vi "Dialog Tester - Preempt.vi"() -> ()   [LabVIEW 2021]
doc: "<b>TEST VI</b> checking the pre-empt action for pop up types"
uses:
  a07ed418-7f18-49d3-b4e5-936e803124ba.vi
  3f576889-9c36-41da-af72-f2da2302e1a7.vi
  ad5c8732-6e62-4ff5-afd9-587a057d3cc7.vi
  5b332a5c-591b-4519-aea1-c482ff36093b.vi
  34588afc-315a-47d8-a701-ee64ae2e0537.vi
  ae7c03dc-1e40-4bc6-b034-dfda178a26ad.vi
  d50a1210-0545-4c1a-9356-5886067c6458.vi
  aeec75d7-a6fb-4d61-b6af-3d1469a3ba41.vi
  6fc38696-eeba-4556-84b5-67169f5a97e1.vi
  54b3774a-3740-4b7d-aaf4-c8348b3dcf84.vi
  f0ad3a18-8d1f-4dec-8074-68e03ac96f8e.vi
  cba20e50-060c-4cef-b2cd-495110a6043b.vi
  Standard/Input (DBL)/Input (DBL).lvclass
  Standard/Input (I32)/Input (I32).lvclass
  Standard/Input (String)/Input (String).lvclass
  Standard/Timeout/Timeout.lvclass
  Standard/Timeout One Button/Timeout One Button.lvclass
  Standard/Timeout Two Button/Timeout Two Button.lvclass
  Standard/Two Button/Two Button.lvclass
  Popup/Popup.lvclass
panel:
  out "Two-Button T.O. Choice? - val":bool
  out "Two-Button Choice? - val":bool
  out "Input Value (String - val)":string
  out "Input Value (I32 - val)":i32
  out "Input Value (DBL - close)":dbl
  out "Two-Button T.O. Choice? - close":bool
  out "Two-Button Choice? - close":bool
  out "Input Value (String - close)":string
  out "Input Value (I32 - close)":i32
  out "Input Value (DBL - val)":dbl
  out "iteration":i32
  in  "Error In":errorcluster
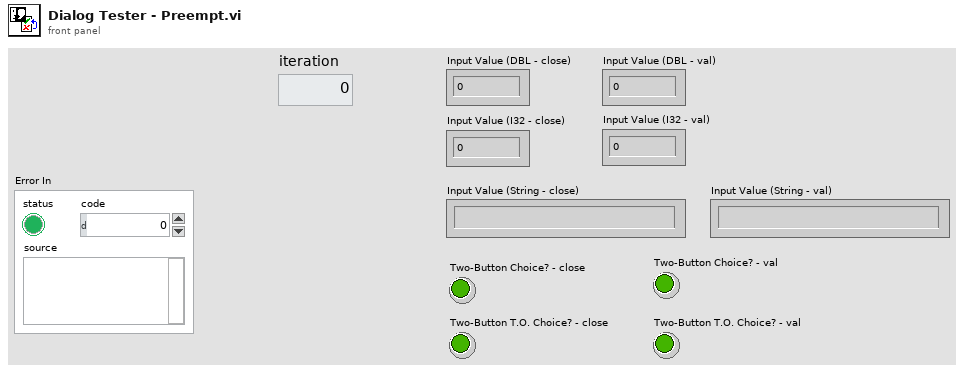
[diagram p1: front panel]
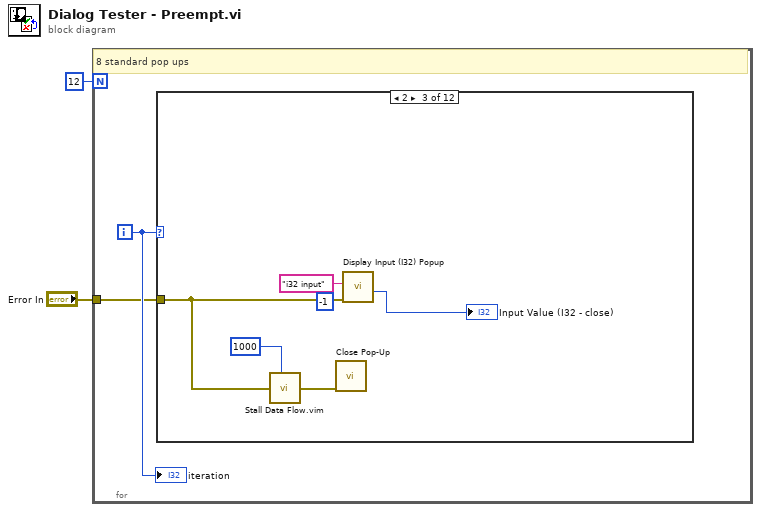
[diagram p0: block diagram]
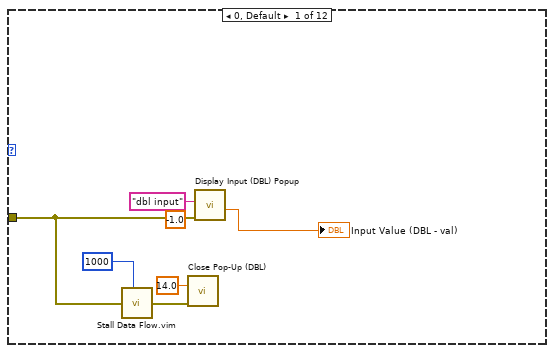
[diagram p2: hidden frame]
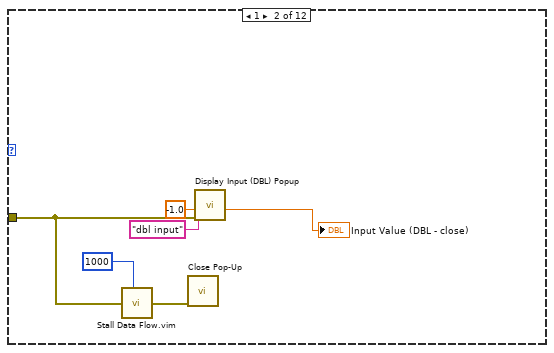
[diagram p3: hidden frame]
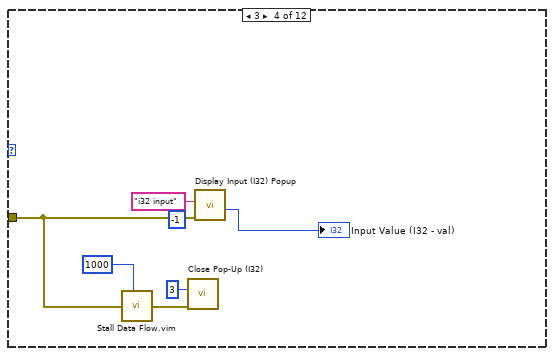
[diagram p4: hidden frame]
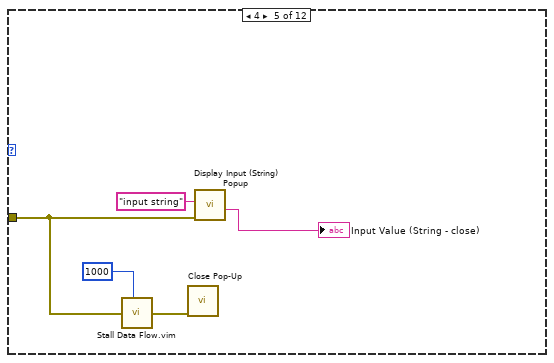
[diagram p5: hidden frame]
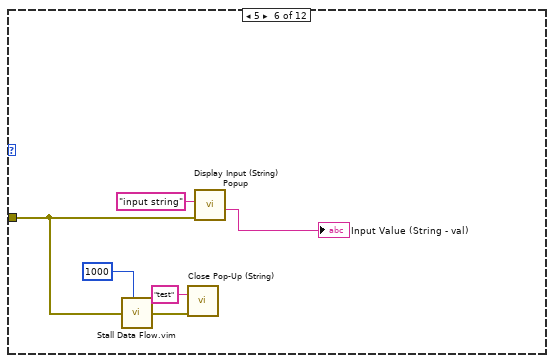
[diagram p6: hidden frame]
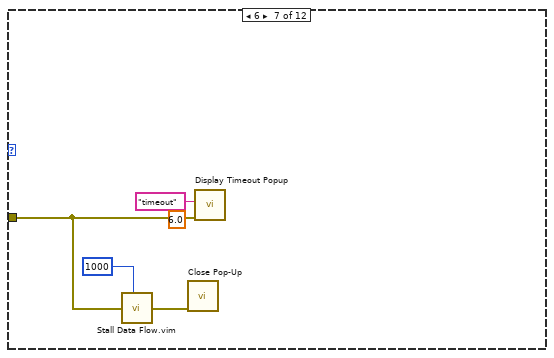
[diagram p7: hidden frame]
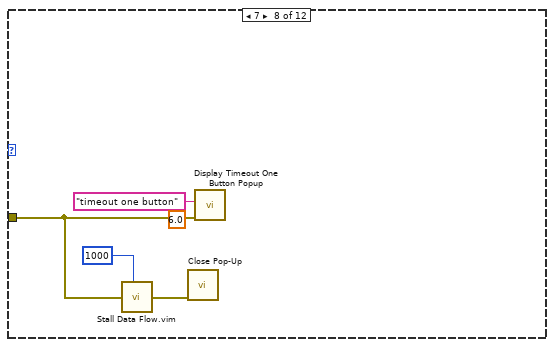
[diagram p8: hidden frame]
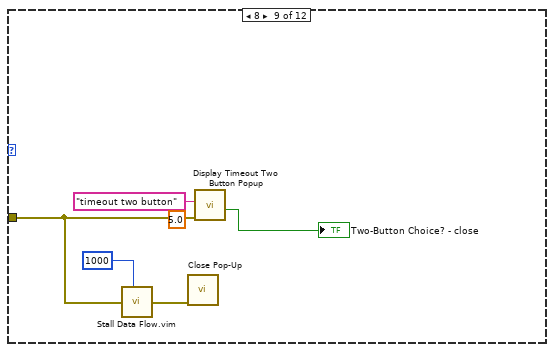
[diagram p9: hidden frame]
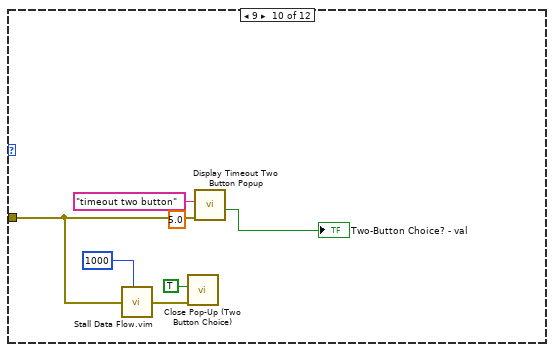
[diagram p10: hidden frame]
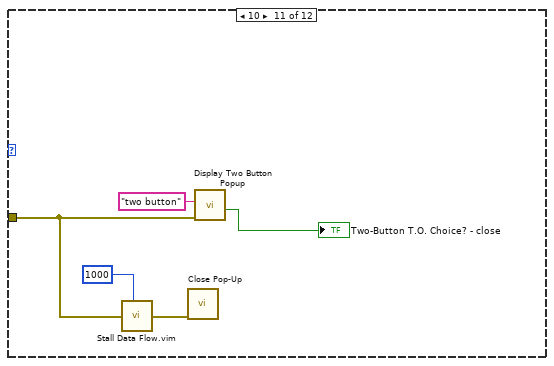
[diagram p11: hidden frame]
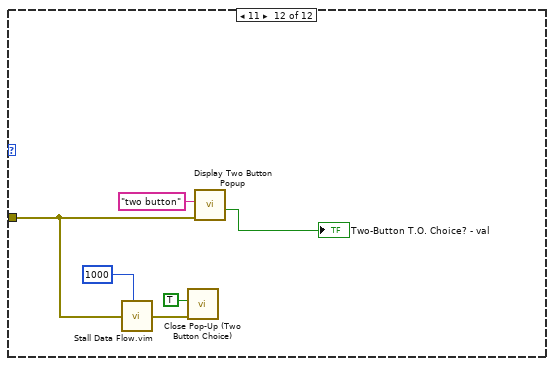
[diagram p12: hidden frame]
diagram:
  n1 = for {
    N: 12 -> [_]
    tunnel: "Error In" -> [w3]
    i -> [w4]
    # "8 standard pop ups"
    n2 = case shown="2" w4 {
      tunnel: w3 -> [w11 w17 w21 w28 w33 w39 w44 w50 w55 w62 w67 w73]
      frame 0, Default {
        n3 = call "Stall Data Flow.vim"("value in"=w11, "milliseconds to wait"=u32 1000) -> ("value out"=w9:errorcluster)  [unwired: 1 out]
        n4 = call "Close Pop-Up (DBL).vi"("error in"=w9, "DBL Default"=14.0) -> ()  [unwired: 9 in, 1 out]
        n5 = call "Display Input (DBL) Popup.vi"("error in"=w11, "Default Input"=-1.0, "Message"="dbl input") -> ("Input Value"=→"Input Value (DBL - val)":dbl)  [unwired: 7 in, 1 out]
      }
      frame 1 {
        n6 = call "Stall Data Flow.vim"("value in"=w17, "milliseconds to wait"=u32 1000) -> ("value out"=w15:errorcluster)  [unwired: 1 out]
        n7 = call "Close Pop-Up.vi"("error in"=w15) -> ()  [unwired: 10 in, 1 out]
        n8 = call "Display Input (DBL) Popup.vi"("error in"=w17, "Default Input"=-1.0, "Message"="dbl input") -> ("Input Value"=→"Input Value (DBL - close)":dbl)  [unwired: 7 in, 1 out]
      }
      frame 2 {
        n9 = call "Stall Data Flow.vim"("value in"=w21, "milliseconds to wait"=u32 1000) -> ("value out"=w22:errorcluster)  [unwired: 1 out]
        n10 = call "Close Pop-Up.vi"("error in"=w22) -> ()  [unwired: 10 in, 1 out]
        n11 = call "Display Input (I32) Popup.vi"("error in"=w21, "Default Input"=-1, "Message"="i32 input") -> ("Input Value"=→"Input Value (I32 - close)":i32)  [unwired: 7 in, 1 out]
      }
      frame 3 {
        n12 = call "Stall Data Flow.vim"("value in"=w28, "milliseconds to wait"=u32 1000) -> ("value out"=w29:errorcluster)  [unwired: 1 out]
        n13 = call "Close Pop-Up (I32).vi"("error in"=w29, "I32 Default"=3) -> ()  [unwired: 9 in, 1 out]
        n14 = call "Display Input (I32) Popup.vi"("error in"=w28, "Default Input"=-1, "Message"="i32 input") -> ("Input Value"=→"Input Value (I32 - val)":i32)  [unwired: 7 in, 1 out]
      }
      frame 4 {
        n15 = call "Stall Data Flow.vim"("value in"=w33, "milliseconds to wait"=u32 1000) -> ("value out"=w34:errorcluster)  [unwired: 1 out]
        n16 = call "Close Pop-Up.vi"("error in"=w34) -> ()  [unwired: 10 in, 1 out]
        n17 = call "Display Input (String) Popup.vi"("error in"=w33, "Message"="input string") -> ("Input Value"=→"Input Value (String - close)":string)  [unwired: 8 in, 1 out]
      }
      frame 5 {
        n18 = call "Stall Data Flow.vim"("value in"=w39, "milliseconds to wait"=u32 1000) -> ("value out"=w40:errorcluster)  [unwired: 1 out]
        n19 = call "Close Pop-Up (String).vi"("error in"=w40, "String Default"="test") -> ()  [unwired: 9 in, 1 out]
        n20 = call "Display Input (String) Popup.vi"("error in"=w39, "Message"="input string") -> ("Input Value"=→"Input Value (String - val)":string)  [unwired: 8 in, 1 out]
      }
      frame 6 {
        n21 = call "Stall Data Flow.vim"("value in"=w44, "milliseconds to wait"=u32 1000) -> ("value out"=w46:errorcluster)  [unwired: 1 out]
        n22 = call "Close Pop-Up.vi"("error in"=w46) -> ()  [unwired: 10 in, 1 out]
        n23 = call "Display Timeout Popup.vi"("error in"=w44, "Timeout (s)"=6.0, "Message"="timeout") -> ()  [unwired: 8 in, 1 out]
      }
      frame 7 {
        n24 = call "Stall Data Flow.vim"("value in"=w50, "milliseconds to wait"=u32 1000) -> ("value out"=w51:errorcluster)  [unwired: 1 out]
        n25 = call "Close Pop-Up.vi"("error in"=w51) -> ()  [unwired: 10 in, 1 out]
        n26 = call "Display Timeout One Button Popup.vi"("error in"=w50, "Timeout (s)"=6.0, "Message"="timeout one button") -> ()  [unwired: 8 in, 1 out]
      }
      frame 8 {
        n27 = call "Stall Data Flow.vim"("value in"=w55, "milliseconds to wait"=u32 1000) -> ("value out"=w56:errorcluster)  [unwired: 1 out]
        n28 = call "Close Pop-Up.vi"("error in"=w56) -> ()  [unwired: 10 in, 1 out]
        n29 = call "Display Timeout Two Button Popup.vi"("error in"=w55, "Timeout (s)"=5.0, "Message"="timeout two button") -> ("Choice"=→"Two-Button Choice? - close":bool)  [unwired: 7 in, 1 out]
      }
      frame 9 {
        n30 = call "Stall Data Flow.vim"("value in"=w62, "milliseconds to wait"=u32 1000) -> ("value out"=w63:errorcluster)  [unwired: 1 out]
        n31 = call "Close Pop-Up (Two Button Choice).vi"("error in"=w63, "Two-Button Choice? (F)"=TRUE) -> ()  [unwired: 9 in, 1 out]
        n32 = call "Display Timeout Two Button Popup.vi"("error in"=w62, "Timeout (s)"=5.0, "Message"="timeout two button") -> ("Choice"=→"Two-Button Choice? - val":bool)  [unwired: 7 in, 1 out]
      }
      frame 10 {
        n33 = call "Stall Data Flow.vim"("value in"=w67, "milliseconds to wait"=u32 1000) -> ("value out"=w68:errorcluster)  [unwired: 1 out]
        n34 = call "Close Pop-Up.vi"("error in"=w68) -> ()  [unwired: 10 in, 1 out]
        n35 = call "Display Two Button Popup.vi"("error in"=w67, "Message"="two button") -> ("Choice"=→"Two-Button T.O. Choice? - close":bool)  [unwired: 8 in, 1 out]
      }
      frame 11 {
        n36 = call "Stall Data Flow.vim"("value in"=w73, "milliseconds to wait"=u32 1000) -> ("value out"=w74:errorcluster)  [unwired: 1 out]
        n37 = call "Close Pop-Up (Two Button Choice).vi"("error in"=w74, "Two-Button Choice? (F)"=TRUE) -> ()  [unwired: 9 in, 1 out]
        n38 = call "Display Two Button Popup.vi"("error in"=w73, "Message"="two button") -> ("Choice"=→"Two-Button T.O. Choice? - val":bool)  [unwired: 8 in, 1 out]
      }
    }
    "iteration" <- w4
  }
